vi "Abort Active DUT SMS.vi"(8 "error in (no error)":errorcluster, 10 "SIM Slot (1)":i32=1, 11 "VISA resource name":refnum<visa-resource-name>) -> (0 "error out":errorcluster, 3 "VISA resource name out":refnum<visa-resource-name>)   [LabVIEW 2020, in "Rohde&Schwarz CMXP Base.lvlib"]
doc: "Cancels the sending of an SMS.\n\nAttributes:\nRSCMXPBASE_ATTR_SELECT_ACTIVE_DUT_SIM_SLOT\nRSCMXPBASE_ATTR_ACTIVE_DUT_SMS_ABORT\n\nRemote-control command:\nABORt:DUT:MODem<ModemIdx>:CONTrol:SMS"
uses:
  <instrlib>/Rohde&Schwarz CMXP Base/Rohde&Schwarz CMXP Base.lvlib
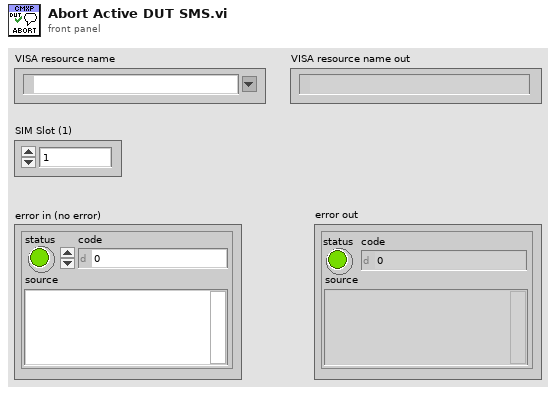
[diagram p1: front panel]
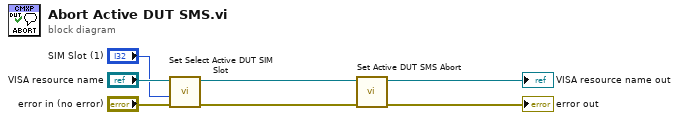
[diagram p0: block diagram]
diagram:
  n1 = call "Set Select Active DUT SIM Slot"("error in (no error)"="error in (no error)", "Select Active DUT SIM Slot (0)"="SIM Slot (1)", "instrument handle"="VISA resource name") -> ("error out"=w4:errorcluster, "instrument handle out"=w5:refnum<visa-resource-name>)  [unwired: 7 in]
  n2 = call "Set Active DUT SMS Abort"("error in (no error)"=w4, "instrument handle"=w5) -> ("error out"=→"error out":errorcluster, "instrument handle out"=→"VISA resource name out":refnum<visa-resource-name>)  [unwired: 8 in]
